vi "Done.vi"(8 "error in (no error)":errorcluster, 11 "ShutdownSink in":refnum<class "Shutdown Sink.lvclass">) -> (0 "error out":errorcluster)   [LabVIEW 2019, in "Network Sink.lvlib" / "Shutdown Sink.lvclass"]
doc: "--\nCopyright © 2017 Composed SystemsI All rights reserved.\n\nAuthor: Jon McBee <jon.mcbee@composed.io>\n\nThis library is provided \"AS IS\" ,WITHOUT WARRANTIES OR\nCONDITIONS OF ANY KIND, either express or implied.\n\nComposed Systems -- composed.io\n\nStream 0.0.1.1\nJon McBee - Composed Systems\nCopyright (c) 2017, Composed Systems"
uses:
  <vilib>/gpm_packages/@cs/event-logger/Source/Network Sink/Shutdown Sink/Shutdown Sink.lvclass
  <vilib>/gpm_packages/@cs/event-logger/Source/Network Sink/Shutdown Sink/Shutdown Sink.lvclass/Shutdown Sink.ctl
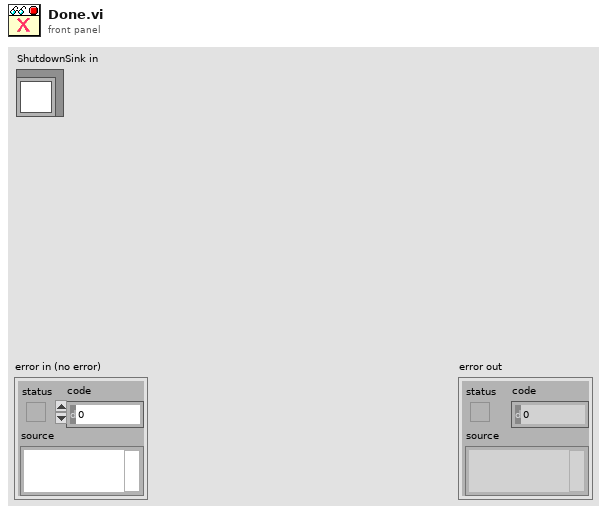
[diagram p1: front panel]
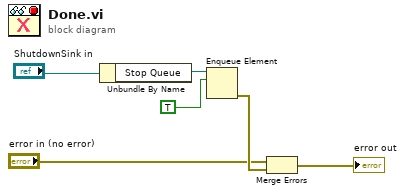
[diagram p0: block diagram]
diagram:
  n1 = Unbundle By Name("ShutdownSink in") -> ("Stop Queue"=w5:refnum<queue>)
  n2 = Enqueue Element(queue=w5, element=TRUE) -> (error out=w4:errorcluster)  [unwired: 2 in, 2 out]
  n3 = Merge Errors("error in (no error)", w4) -> (→"error out":errorcluster)
